vi "DataProcessorDEMBUT.vi"(4 "Settling":enum16{"99%", "99,9%"}(ring)=enum."99,9%", 6 "Filter Order":u32=1 min=1 max=4, 8 "FPGA in":refnum<queue>, 11 "DATA in":refnum<queue>) -> ()   [LabVIEW 2019, in "FPGA.lvlib"]
uses:
  FPGA.lvlib
  FPGA.ctl
  <vilib>/Analysis/1siggen.llb/Ramp Pattern by Samples.vi
  ResultSweep.vi
  <vilib>/Analysis/NI_AALBase.lvlib
panel:
  in  "Save raw data":bool
  in  "Store raw data":bool
  out "Raw Data Quadrature":dbl[](graph)
  out "Raw Data Phase":dbl[](graph)
  out "Module":cluster{dbl[], dbl[]}(graph)
  out "Phase":cluster{dbl[], dbl[]}(graph)
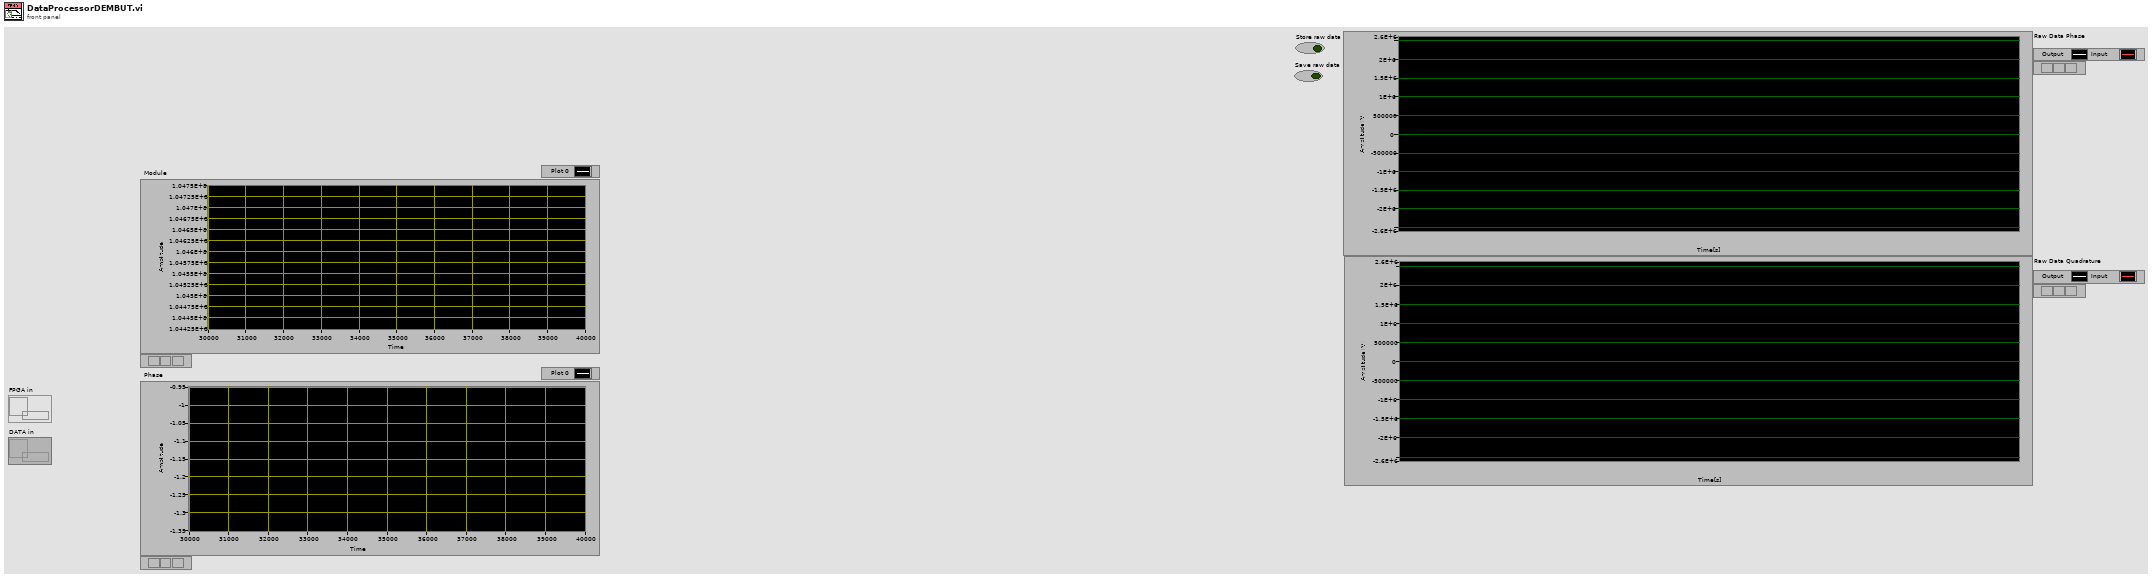
[diagram p1: front panel]
types:
  T1 = typedef "FPGA.lvlib/FPGA.ctl" = cluster{"Start freq. [Hz]":dbl, "Sweep duration [s]":dbl, "Freq. step [Hz]":dbl, "DAC Sample Rate":dbl, "ADC Sample Rate":dbl, "CMD port":u16, "DFAST port":u16, "CMD ID":refnum<k16>, "DFAST ID":refnum<k16>, "CMD error out":errorcluster, "FPGA IP":string, "DFAST error out ":errorcluster, "Stop freq. [Hz]":dbl, "Discrete sweep":bool, "Initial NCO":u32, "Difference NCO":i32, "step NCO":i64, "Final NCO":u32, "clocks for step":u32, "demodulation":bool, "NCO Phase Precision":u32, "NCO Sample Rate":dbl, "Time for step [s]":dbl, "NCO freq. resolution":dbl, "Sweep speed [Hz/s]":dbl, "Connected":bool, "Slew Rate [V/us]":dbl, "Parameters_ok":bool, "Amplitude [mVpp]":dbl, "Scale Factor":fxp<+,16,0>, "Acquiring":bool, "DAC-ADC Latency":u16, "Digital Gain":i32, "Number of steps":i32, "Averaging preferred":bool, "Filter Order":u32, "Settling":enum16{"99%", "99,9%"}, "FIFO":cluster{"Start freq. [Hz]":dbl, "Sweep duration [s]":dbl, "Freq. step [Hz]":dbl, "Stop freq. [Hz]":dbl, "Time for step [s]":dbl, "Amplitude [mVpp]":dbl, "Number of steps":i32}[]}
  T2 = cluster{"filter structure":enum32{"IIR 2nd Order", "IIR 4th Order"}, "Reverse Coefficients":dbl[], "Forward Coefficients":dbl[]}
  T3 = cluster{"Name":string, "Color":u32, "Style":u8, "Point Style":u8, "Name Visible":bool, "Allow Drag":bool, "Cursor Mode":u32, "Plot":i32, "Index":i32, "Position":cluster{"X":dbl, "Y":dbl}, "X Scale":u32, "Y Scale":u32, "Watch Plots":i32[], "Watch All Plots":bool, "Plot Area":i32, "Label Offset":cluster{"X":dbl, "Y":dbl}}
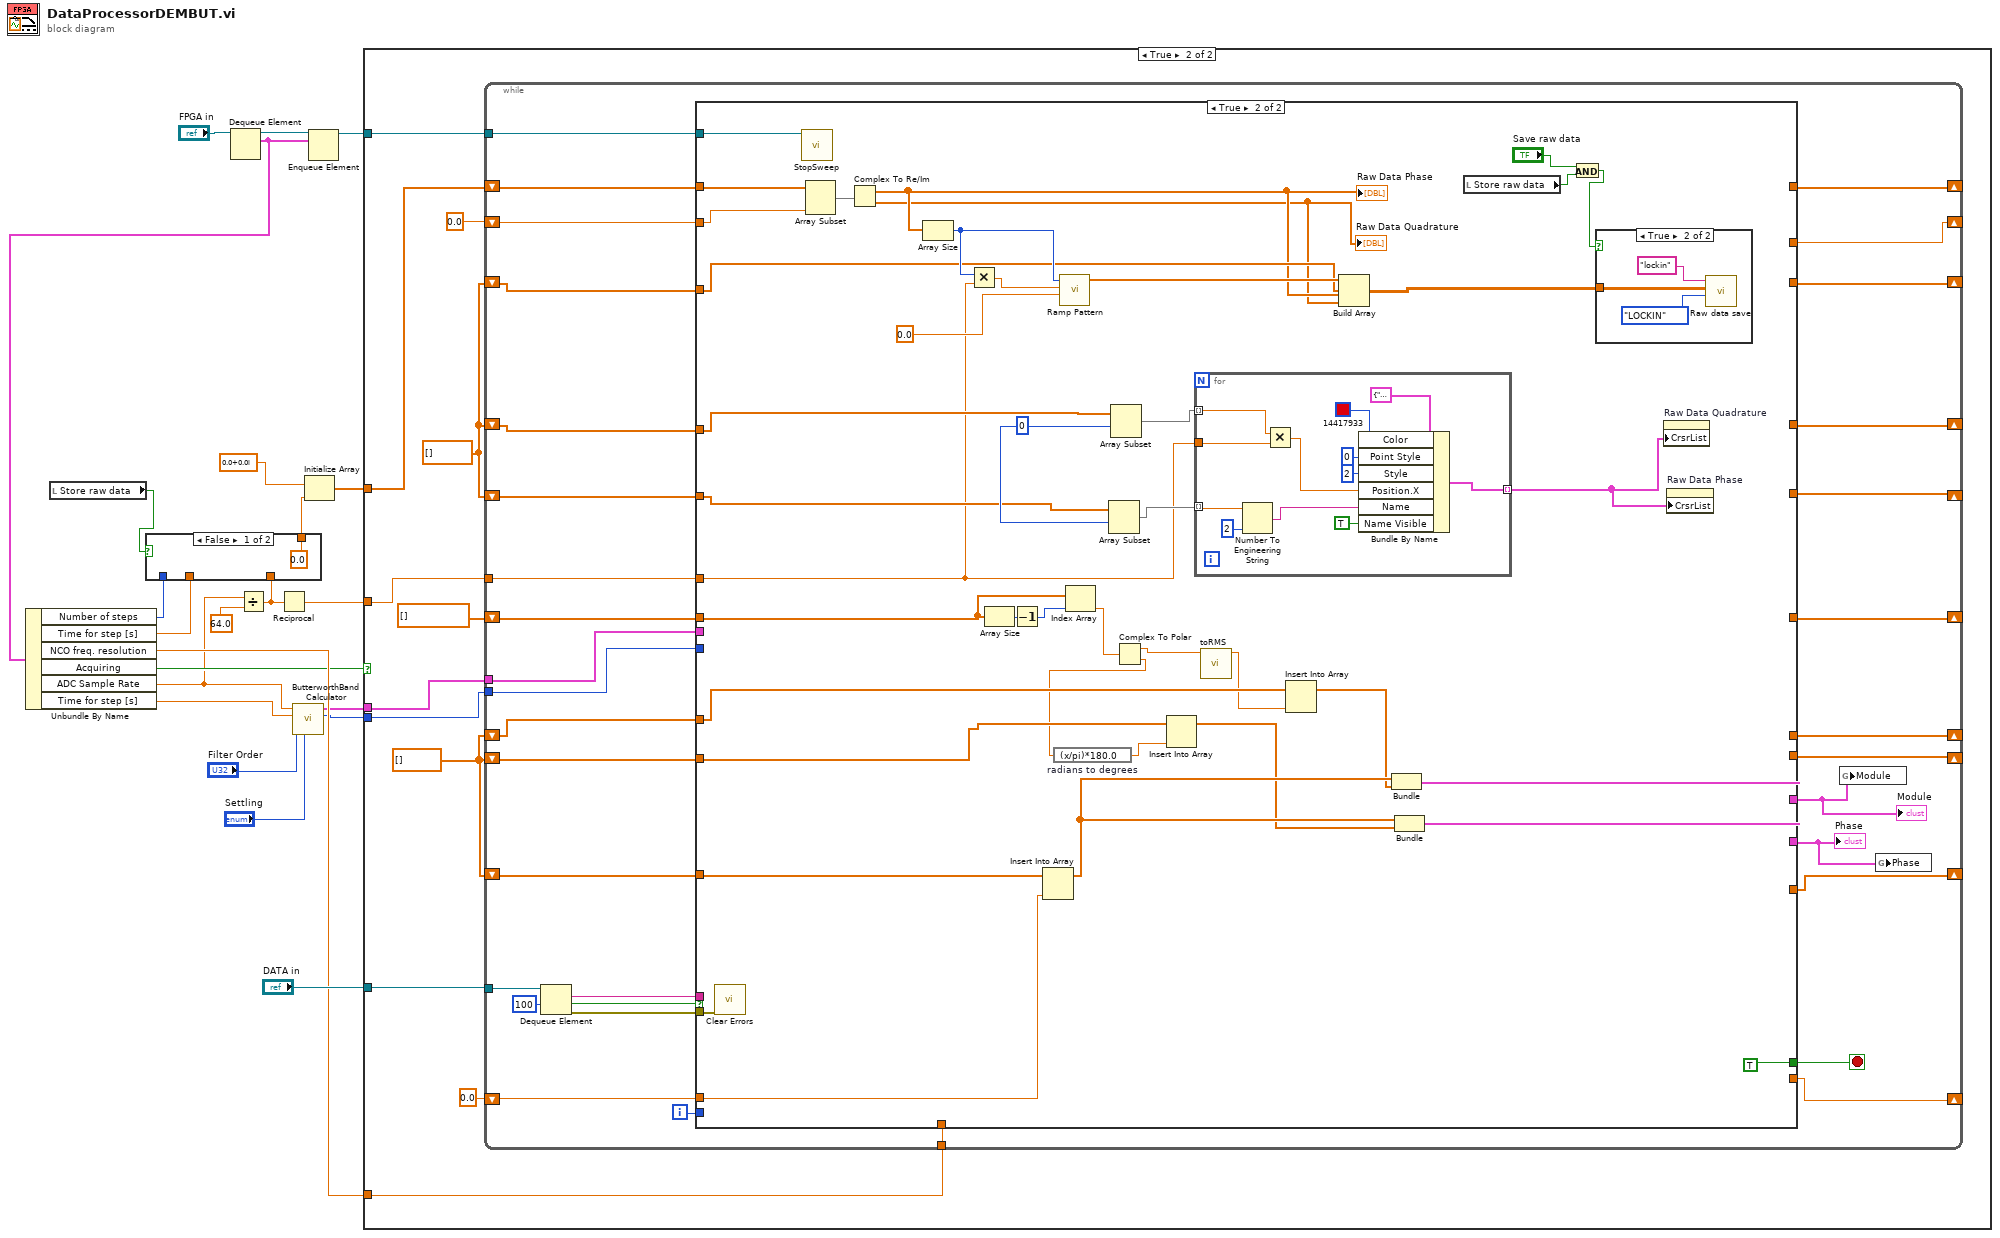
[diagram p0: block diagram]
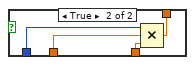
[diagram p2: hidden frame]
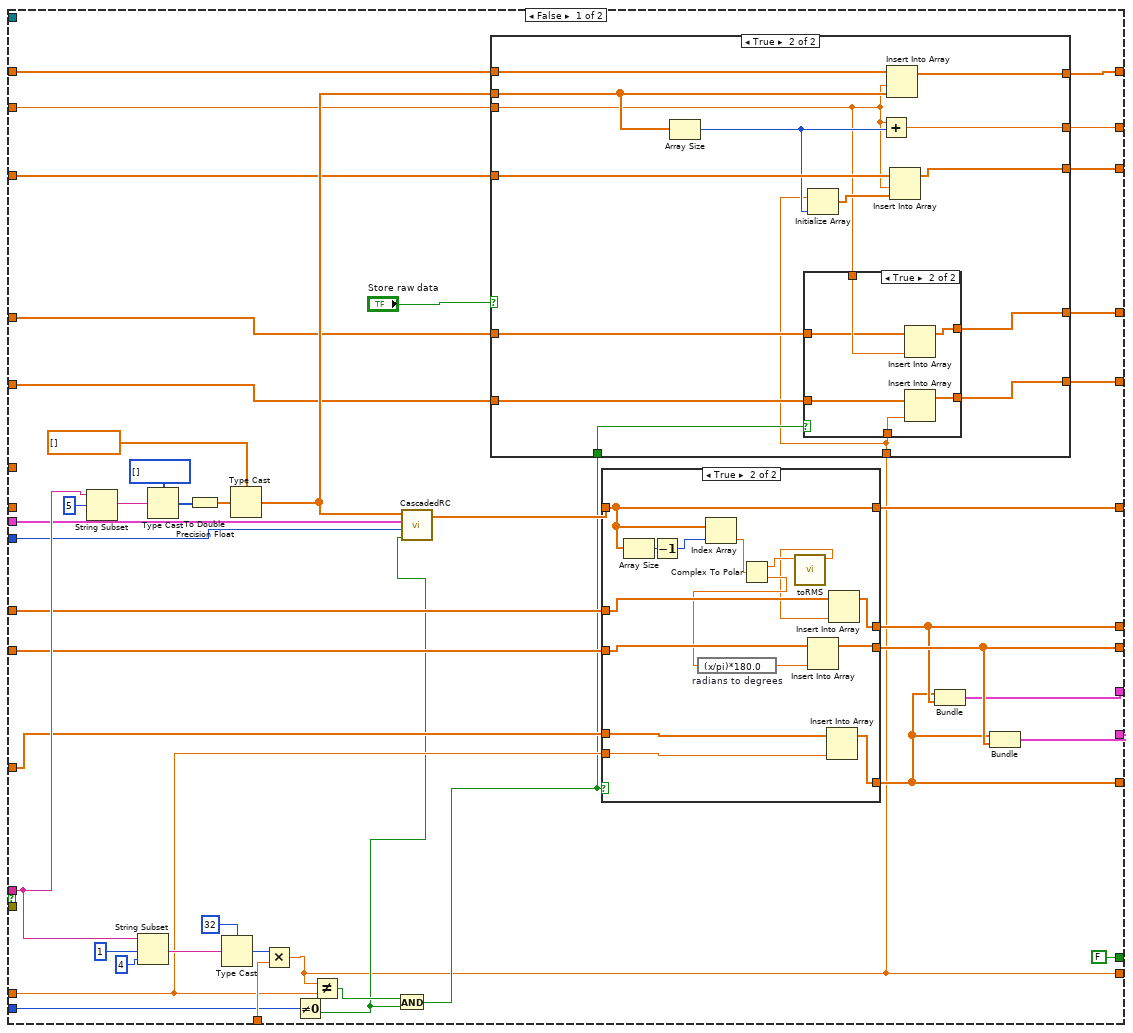
[diagram p4: hidden frame]
diagram:
  n1 = local read "Store raw data"() -> (w1:bool)
  n2 = Dequeue Element(queue="FPGA in") -> (queue out=w18:refnum<queue>, element=w17:T1)  [unwired: 2 in, 2 out]
  n3 = Unbundle By Name(w17) -> ("Number of steps"=w2:i32, "Time for step [s]"=w8:dbl, "NCO freq. resolution"=w20:dbl, "Acquiring"=w19:bool, "ADC Sample Rate"=w9:dbl, "Time for step [s]"=w15:dbl)
  n4 = Divide(x=w9, y=64.0) -> (x/y=w4:dbl)
  n5 = case shown="False" w1 {
    tunnel: w8 -> [_ w27]
    tunnel: [0.0 w26] -> w7
    tunnel: w4 -> [_ w25]
    tunnel: w2 -> [_ w24]
    frame False {
    }
    frame True {
      n6 = Compound Arithmetic op=MULTIPLY(w24, w27, w25) -> (w26:dbl)
    }
  }
  n7 = Reciprocal(x=w4) -> (1/x=w3:dbl)
  n8 = call "ButterworthBandCalculator.vi"("Settling"="Settling", "Filter Order"="Filter Order", "Regime time"=w15, "ADC Sample Rate"=w9) -> ("N. stages"=w12:u32, "IIR Filter out"=w14:T2)  [unwired: 3 in, 3 out]
  n9 = Initialize Array(cdb 0.0+0.0i, w7) -> (w5:cdb[])
  n10 = Enqueue Element(queue=w18, element=w17) -> (queue out=w16:refnum<queue>)  [unwired: 2 in, 2 out]
  n11 = case shown="True" w19 {
    tunnel: w20 -> [_ w38]
    tunnel: "DATA in" -> [_ w39]
    tunnel: w16 -> [_ w36]
    tunnel: w14 -> [_ w33]
    tunnel: w12 -> [_ w32]
    tunnel: w5 -> [_ w31]
    tunnel: w3 -> [_ w29]
    frame False {
    }
    frame True {
      w28 = dbl[] []
      w35 = dbl[] []
      n12 = while {
        tunnel: w39 -> [w72]
        shift-right: [w67] -> _
        shift-left: 0.0 ("length (rest)") -> [w68]
        tunnel: w38 -> [w69]
        shift-right: [w65] -> _
        shift-left: w35 -> [w66]
        shift-right: [w62] -> _
        shift-left: w35 -> [w63]
        tunnel: w36 -> [w61]
        shift-right: [w59] -> _
        shift-left: w35 -> [w60]
        shift-right: [w54] -> _
        shift-left: w31 -> [w55]
        shift-right: [w52] -> _
        shift-left: cdb[] [] -> [w51]
        tunnel: w33 -> [w50]
        tunnel: w32 -> [w49]
        shift-right: [w47] -> _
        shift-left: 0.0 ("mean") -> [w48]
        shift-right: [w43] -> _
        shift-left: w28 -> [w44]
        shift-right: [w45] -> _
        shift-left: w28 -> [w46]
        tunnel: w29 -> [w42]
        shift-right: [w40] -> _
        shift-left: w28 -> [w41]
        i -> [w64]
        stop <- w53 stop-if-true
        n13 = Dequeue Element(queue=w72, timeout in ms (-1)=100) -> (element=w71:string, timed out?=w58:bool, error out=w70:errorcluster)  [unwired: 1 in, 1 out]
        n14 = case shown="True" w58 {
          tunnel: w71 -> [w115 _]
          tunnel: w70 -> [_ w205]
          tunnel: w69 -> [w112 _]
          tunnel: w68 -> [w107 w203]
          tunnel: [w81 _] -> w67
          tunnel: w66 -> [w111 w192]
          tunnel: [w99 _] -> w65
          tunnel: w64 -> [w91 _]
          tunnel: w63 -> [w108 w204]
          tunnel: [w95 _] -> w62
          tunnel: w61 -> [_ w202]
          tunnel: w60 -> [w100 w193]
          tunnel: [w97 _] -> w59
          tunnel: [w96 w201] -> w57
          tunnel: [w98 w200] -> w56
          tunnel: w55 -> [w94 w187]
          tunnel: [w93 _] -> w54
          tunnel: [FALSE TRUE] -> w53
          tunnel: [w92 _] -> w52
          tunnel: w51 -> [_ w194]
          tunnel: w50 -> [w90 _]
          tunnel: w49 -> [w89 _]
          tunnel: w48 -> [w84 w186]
          tunnel: [w83 _] -> w47
          tunnel: w46 -> [w80 w181]
          tunnel: [w79 _] -> w45
          tunnel: w44 -> [w78 w180]
          tunnel: [w77 _] -> w43
          tunnel: w42 -> [_ w177]
          tunnel: w41 -> [w75 w173]
          tunnel: [w74 _] -> w40
          frame False {
            n15 = String Subset(string=w115, offset (0)=5) -> (substring=w101:string)  [unwired: 1 in]
            n16 = String Subset(string=w115, offset (0)=1, length (rest)=4 ("length (rest)")) -> (substring=w114:string)
            n17 = Type Cast(type=i32[] [], x=w101) -> (*(type *) &x=w105:i32[])
            n18 = To Double Precision Float(number=w105) -> (double precision float=w104:dbl[])
            n19 = Type Cast(type=u32 32 ("length (rest)"), x=w114) -> (*(type *) &x=w110:u32)
            n20 = Type Cast(type=cdb[] [], x=w104) -> (*(type *) &x=w86:cdb[])
            n21 = Multiply(x=w110, y=w112) -> (x*y=w81:dbl)
            n22 = Not Equal To 0?(x=w91) -> (x != 0?=w88:bool)
            n23 = Not Equal?(x=w81, y=w107) -> (x != y?=w109:bool)
            n24 = And(x=w109, y=w88) -> (x .and. y?=w82:bool)
            n25 = call "CascadedRC.vi"("init/cont (init:F)"=w88, "N. stages"=w89, "IIR Filter in"=w90, "X"=w86) -> ("Filtered X"=w87:cdb[])  [unwired: 7 in]
            n26 = case shown="True" "Store raw data" {
              tunnel: w94 -> [w122 w137]
              tunnel: [w122 w136] -> w93
              tunnel: w86 -> [_ w135]
              tunnel: w84 -> [w121 w124]
              tunnel: [w121 w134] -> w83
              tunnel: w82 -> [_ w133]
              tunnel: w81 -> [_ w123]
              tunnel: w80 -> [w119 w132]
              tunnel: [w119 w131] -> w79
              tunnel: w78 -> [w120 w130]
              tunnel: [w120 w129] -> w77
              tunnel: w75 -> [w118 w128]
              tunnel: [w118 w127] -> w74
              frame False {
              }
              frame True {
                n27 = Array Size(array=w135) -> (size(s)=w126:i32)
                n28 = case shown="True" w133 {
                  tunnel: w124 -> [_ w145]
                  tunnel: w123 -> [_ w140]
                  tunnel: w132 -> [w138 w144]
                  tunnel: [w138 w143] -> w131
                  tunnel: w130 -> [w139 w142]
                  tunnel: [w139 w141] -> w129
                  frame False {
                  }
                  frame True {
                    n29 = Insert Into Array(array=w142, new element=w145) -> (w141:dbl[])  [unwired: 1 in]
                    n30 = Insert Into Array(array=w144, new element=w140) -> (w143:dbl[])  [unwired: 1 in]
                  }
                }
                n31 = Initialize Array(w123, w126) -> (w125:dbl[])
                n32 = Add(x=w124, y=w126) -> (x+y=w134:dbl)
                n33 = Insert Into Array(array=w137, index=w124, new element=w135) -> (w136:cdb[])
                n34 = Insert Into Array(array=w128, index=w124, new element=w125) -> (w127:dbl[])
              }
            }
            n35 = case shown="True" w82 {
              tunnel: w111 -> [w149 w157]
              tunnel: [w149 w156] -> w99
              tunnel: w108 -> [w148 w164]
              tunnel: [w148 w162] -> w95
              tunnel: w107 -> [_ w163]
              tunnel: w100 -> [w147 w159]
              tunnel: [w147 w158] -> w97
              tunnel: w87 -> [w146 w154]
              tunnel: [w146 w154] -> w92
              frame False {
              }
              frame True {
                n36 = Array Size(array=w154) -> (size(s)=w161:i32)
                n37 = Decrement(x=w161) -> (x-1=w160:i32)
                n38 = Index Array(array=w154, index=w160) -> (element=w155:cdb)
                n39 = Complex To Polar(r * e^(i*theta)=w155) -> (r=w151:dbl, theta=w152:dbl)
                n40 = expression code="(x/pi)*180.0" "radians to degrees"(w152) -> (w153:dbl)
                n41 = call "toRMS.vi"("Input"=w151) -> ("Output [Vrms]"=w150:dbl)  [unwired: 10 in]
                n42 = Insert Into Array(array=w157, new element=w153) -> (w156:dbl[])  [unwired: 1 in]
                n43 = Insert Into Array(array=w164, new element=w163) -> (w162:dbl[])  [unwired: 1 in]
                n44 = Insert Into Array(array=w159, new element=w150) -> (w158:dbl[])  [unwired: 1 in]
              }
            }
            n45 = Bundle(w95, w97) -> (w96:cluster{dbl[], dbl[]})  [unwired: 1 in]
            n46 = Bundle(w95, w99) -> (w98:cluster{dbl[], dbl[]})  [unwired: 1 in]
          }
          frame True {
            w183 = 0 ("index")
            n47 = call <vilib>:"Clear Errors.vi"("error in (no error)"=w205) -> ()  [unwired: 5 in, 2 out]
            n48 = call "StopSweep.vi"("FPGA in"=w202) -> ()  [unwired: 10 in, 1 out]
            n49 = Array Subset(array=w187, length=w186) -> (w185:cdb[])  [unwired: 1 in]
            n50 = Complex To Re/Im(x + iy=w185) -> (x=w172:dbl[], y=w171:dbl[])
            "Raw Data Phase" <- w172
            "Raw Data Quadrature" <- w171
            n51 = Array Size(array=w172) -> (size(s)=w175:i32)
            n52 = Multiply(x=w175, y=w177) -> (x*y=w176:dbl)
            n53 = Array Size(array=w194) -> (size(s)=w197:i32)
            n54 = Decrement(x=w197) -> (x-1=w196:i32)
            n55 = Insert Into Array(array=w204, new element=w203) -> (w199:dbl[])  [unwired: 1 in]
            n56 = call-poly <vilib>:"Ramp Pattern.vi"("start"=0.0, "end"=w176, "samples"=w175) -> ("Ramp Pattern"=w174:dbl[])  [unwired: 7 in, 1 out]
            n57 = Index Array(array=w194, index=w196) -> (element=w195:cdb)
            n58 = Array Subset(array=w181, index=w183) -> (w184:dbl[])  [unwired: 1 in]
            n59 = Array Subset(array=w180, index=w183) -> (w182:dbl[])  [unwired: 1 in]
            n60 = Complex To Polar(r * e^(i*theta)=w195) -> (r=w166:dbl, theta=w188:dbl)
            n61 = expression code="(x/pi)*180.0" "radians to degrees"(w188) -> (w189:dbl)
            n62 = Insert Into Array(array=w192, new element=w189) -> (w191:dbl[])  [unwired: 1 in]
            n63 = for {
              tunnel: [w220] -> w179 mode=indexing
              tunnel: w182 -> [w217] mode=indexing
              tunnel: w177 -> [w218]
              tunnel: w184 -> [w212] mode=indexing
              n64 = Number To Engineering String(2:i16 2 ("precision (6)"), 4:w212) -> (0:w211:string)  [unwired: 2 in]
              n65 = Multiply(x=w217, y=w218) -> (x*y=w216:dbl)
              n66 = Bundle By Name(cluster=T3 {"Name"="", "Color"=0, "Style"=0, "Point Style"=0, "Name Visible"=FALSE, "Allow Drag"=FALSE, "Cursor Mode"=0, "Plot"=0, "Index"=0, "Position"={"X"=0.0, "Y"=0.0}, "X Scale"=0, "Y Scale"=0, "Watch Plots"=[], "Watch All Plots"=FALSE, "Plot Area"=0, "Label Offset"={"X"=0.0, "Y"=0.0}}, "Color"=u32 14417933, "Point Style"=u8 0, "Style"=u8 2, "Position.X"=w216, "Name"=w211, "Name Visible"=TRUE) -> (w220:T3)
            }
            n67 = call "toRMS.vi"("Input"=w166) -> ("Output [Vrms]"=w165:dbl)  [unwired: 10 in]
            n68 = Insert Into Array(array=w193, new element=w165) -> (w190:dbl[])  [unwired: 1 in]
            n69 = Build Array(w174, w173, w172, w171) -> (w167:dbl[][])
            n70 = Bundle(w199, w190) -> (w201:cluster{dbl[], dbl[]})  [unwired: 1 in]
            n71 = Bundle(w199, w191) -> (w200:cluster{dbl[], dbl[]})  [unwired: 1 in]
            n72 = local read "Store raw data"() -> (w170:bool)
            n73 = And(x="Save raw data", y=w170) -> (x .and. y?=w168:bool)
            n74 = case shown="True" w168 {
              tunnel: w167 -> [_ w208]
              frame False {
              }
              frame True {
                n75 = call "Raw data save.vi"("Enum"=enum16{"LOCKIN", "RAW"}."LOCKIN", "Input"=w208, "file format"="lockin") -> ()  [unwired: 9 in]
              }
            }
            n76 = property on="Raw Data Quadrature" class="WFGraph (strict)"("CrsrList"=w179) -> ()  [unwired: 2 in, 2 out]
            n77 = property on="Raw Data Phase" class="WFGraph (strict)"("CrsrList"=w179) -> ()  [unwired: 2 in, 2 out]
          }
        }
        "Module" <- w57
        "Phase" <- w56
        n78 = global write "ResultSweep.vi" "Module"(w57) -> ()
        n79 = global write "ResultSweep.vi" "Phase"(w56) -> ()
      }
    }
  }
